vi "SPI API - SPI Simulation.vi"() -> ()   [LabVIEW 2014]
uses:
  Controls/Digital Data.ctl
  <vilib>/rvi/DesktopExecutionNode/DesktopExecutionNode.xnode
  <userlib>/_NI SPI IP/FPGA/Controllers/Public/Transfer Settings.ctl
  <userlib>/_NI SPI IP/FPGA/Controllers/NI SPI IP FPGA.lvlib
  <vilib>/rvi/DesktopExecutionNode/Execution/niFpgaDEN_Execute.vi
  Controls/Timing Characteristics.ctl
panel:
  out "Data To Slave":u64 format="%b"
  out "Timing Characteristics":T1 {"tCL (ns)" format="%#_4g"; "tCH (ns)" format="%#_4g"; "tCP (ns)" format="%#_4g"; "tCSS (ns)" format="%#_4g"; "tCSH (ns)" format="%#_4g"; "tCSW (ns)" format="%#_4g"; "Actual Sample Rate (Hz)" format="%_4p"; "SCLK Frequency (Hz)" format="%#.2p"}
  in  "Pause":bool
  in  "Sample Rate (Hz)":u32=75000
  out "Digital Data":digitalwaveform(graph)
  in  "Data To Slave":u64
  in  "Stop":bool
  # "Operating Instructions\n1. For this VI to work, the FPGA must be in Simulation Mode.\n2. Run the VI and change the 'SPI PHY Settings' and 'Data To Slave' controls to change the SPI Output.\n3. While changing the settings, view the timing characteristics of the signal on the right side of the graph."
  # "Typical Timing Diagram"
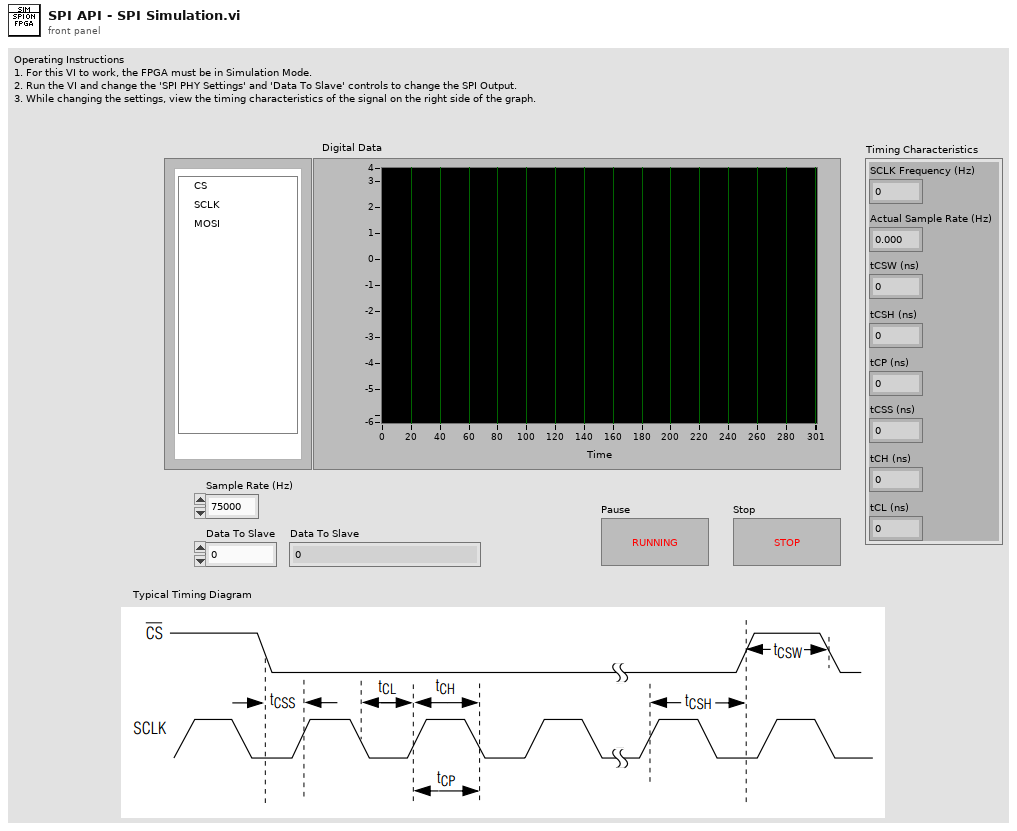
[diagram p1: front panel]
types:
  T1 = typedef "Timing Characteristics.ctl" = cluster{"SCLK Frequency (Hz)":dbl, "Actual Sample Rate (Hz)":dbl, "tCSW (ns)":dbl, "tCSH (ns)":dbl, "tCSS (ns)":dbl, "tCP (ns)":dbl, "tCH (ns)":dbl, "tCL (ns)":dbl}
  T2 = typedef "NI SPI IP FPGA.lvlib/Transfer Settings.ctl" = cluster{"Divide Value":u8, "Transfer Length (bits)":u8, "CS Asserted Polarity":bool, "Clock Polarity (CPOL)":bool, "Clock Phase (CPHA)":bool, "Lengthen MISO Setup":bool, "Direction Change Bit":u8, "MOSI Starts as Output":bool, "Tristatable MOSI":bool}
  T3 = typedef "Digital Data.ctl" = cluster{"CS":bool, "SCLK":bool, "MISO":bool}
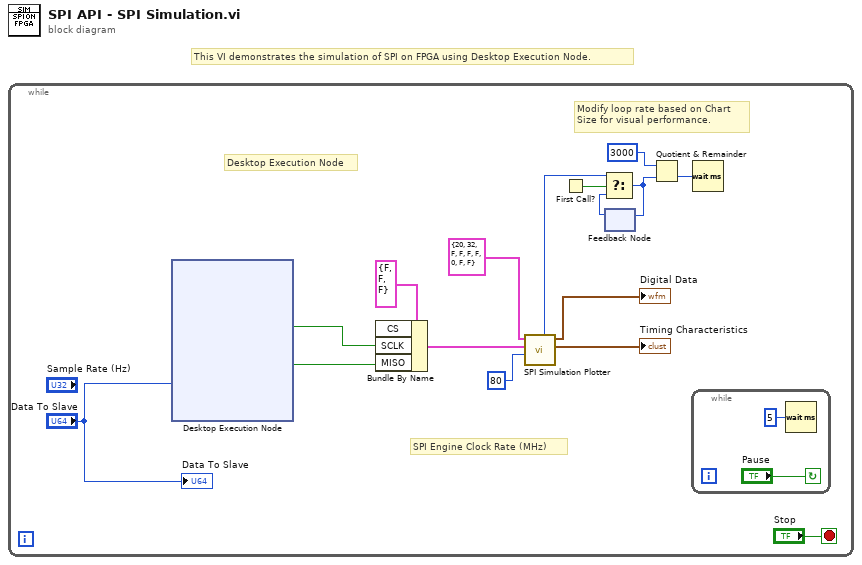
[diagram p0: block diagram]
diagram:
  # "This VI demonstrates the simulation of SPI on FPGA using Desktop Execution Node."
  n1 = while {
    stop <- "Stop" stop-if-true
    # "Desktop Execution Node"
    # "SPI Engine Clock Rate (MHz)"
    # "Modify loop rate based on Chart\nSize for visual performance."
    n2 = xnode "Desktop Execution Node"("Tx"="Data To Slave") -> ("CS"=w4:bool, "MOSI"=w3:bool)  [unwired: 2 in, 2 out]
    n3 = Bundle By Name(cluster=T3 {"CS"=FALSE, "SCLK"=FALSE, "MISO"=FALSE}, "SCLK"=w4, "MISO"=w3) -> (w9:T3)  [unwired: 1 in]
    n4 = call "SPI Simulation Plotter.vi"("Engine Clock Rate (MHz)"=80, "SPI Signals"=w9, "SPI PHY Settings"=T2 {"Divide Value"=20, "Transfer Length (bits)"=32, "CS Asserted Polarity"=FALSE, "Clock Polarity (CPOL)"=FALSE, "Clock Phase (CPHA)"=FALSE, "Lengthen MISO Setup"=FALSE, "Direction Change Bit"=0, "MOSI Starts as Output"=FALSE, "Tristatable MOSI"=FALSE}) -> ("Timing Characteristics"=→"Timing Characteristics":T1, "Digital Data"=→"Digital Data":digitalwaveform, "Chart Size"=w8:i32)  [unwired: 6 in]
    n5 = First Call?() -> (First Call?: T/F=w14:bool)
    n6 = feedback #1() -> (w13:i32)  [unwired: 1 in]
    n7 = Select(t=w8, s=w14, f=w13) -> (s? t:f=w12:i32)
    n8 = feedback-in #1(w12) -> ()
    n9 = Quotient & Remainder(x=u32 3000 ("ms per Command"), y=w12) -> (floor(x/y)=w10:u32)  [unwired: 1 out]
    n10 = while {
      stop <- "Pause" continue-if-true
      n11 = Wait (ms)(milliseconds to wait=u32 5) -> ()  [unwired: 1 out]
    }
    n12 = Wait (ms)(milliseconds to wait=w10) -> ()  [unwired: 1 out]
    "Data To Slave" <- "Data To Slave"
  }
